vi "read_ini_file.vi"(8 "error in (no error)":errorcluster, 11 "configuration file path":path=path "D:/config.ini") -> (0 "error out":errorcluster, 1 "values":string[](array[string]), 2 "keys":string[](array[string]), 3 "sections":string[](array[string]))   [LabVIEW 2009]
uses:
  <vilib>/Utility/config.llb/Read Key (String).vi
  <vilib>/Utility/config.llb/NI_LVConfig.lvlib
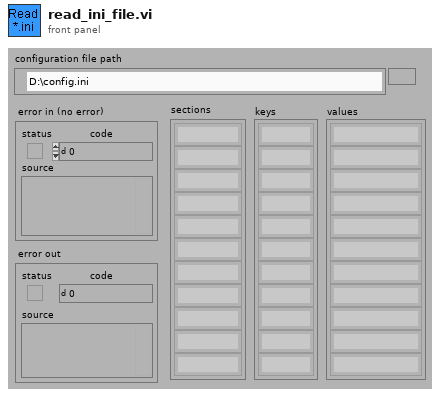
[diagram p1: front panel]
types:
  T1 = typedef "NI_LVConfig.lvlib/Config Data RefNum.ctl" = refnum<k1>
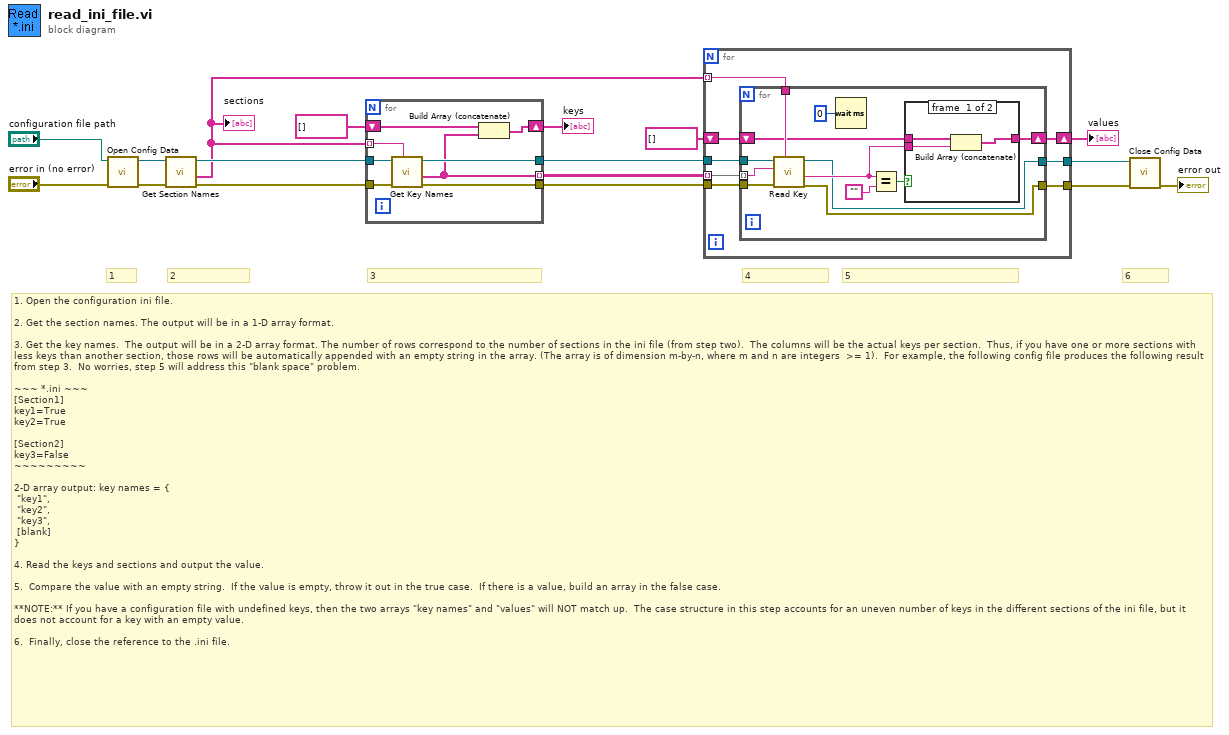
[diagram p0: block diagram]
diagram:
  # "1. Open the configuration ini file.\n\n2. Get the section names. The output will be in a 1-D array format.\n\n3. Get the key names.  The output will be in a 2-D array format. The number of rows correspond to the number of sections in the ini file (from step two).  The columns will be the actual keys per section.  Thus, if you have one or more sections with less keys than another section, those rows will be automatically appended with an empty string in the array. (The array is of dimension m-by-n, where m and n are integers  >= 1).  For example, the following config file produces the following result from step 3.  No worries, step 5 will address this \"blank space\" problem.\n\n~~~ *.ini ~~~\n[Section1]\nkey1=True\nkey2=True\n\n[Section2]\nkey3=False\n~~~~~~~~~\n\n2-D array output: key names = {\n \"key1\",\n \"key2\",\n \"key3\",\n [blank]\n}\n\n4. Read the keys and sections and output the value.\n\n5.  Compare the value with an empty string.  If the value is empty, throw it out in the true case.  If there is a value, build an array in the false case.\n\n**NOTE:** If you have a configuration file with undefined keys, then the two arrays \"key names\" and \"values\" will NOT match up.  The case structure in this step accounts for an uneven number of keys in the different sections of the ini file, but it does not account for a key with an empty value.\n\n6.  Finally, close the reference to the .ini file."
  # "6"
  # "5"
  # "4"
  # "3"
  # "2"
  # "1"
  n1 = call <vilib>:"Open Config Data.vi"("error in (no error)"="error in (no error)", "configuration file path"="configuration file path") -> ("error out"=w17:errorcluster, "refnum"=w16:T1)  [unwired: 7 in, 1 out]
  n2 = call <vilib>:"Get Section Names.vi"("error in (no error)"=w17, "refnum"=w16) -> ("error out"=w14:errorcluster, "section names"=w8:string[], "refnum out"=w15:T1)  [unwired: 7 in]
  "sections" <- w8
  n3 = for {
    tunnel: w15 -> [w25]
    tunnel: w14 -> [w24]
    tunnel: [w23] -> w9
    tunnel: [w22] -> w10
    tunnel: w8 -> [w21] mode=indexing
    shift-right: [w20] -> w6
    shift-left: string[] [] -> [w19]
    tunnel: [w18] -> w5 mode=indexing
    n4 = call <vilib>:"Get Key Names.vi"("section"=w21, "error in (no error)"=w24, "refnum"=w25) -> ("error out"=w23:errorcluster, "key names"=w18:string[], "refnum out"=w22:T1)  [unwired: 5 in, 1 out]
    n5 = Build Array (concatenate)(w19, w18) -> (w20:string[])
  }
  "keys" <- w6
  n6 = for {
    tunnel: w10 -> [w32]
    tunnel: w9 -> [w33]
    tunnel: w8 -> [w31] mode=indexing
    tunnel: w5 -> [w30] mode=indexing
    shift-right: [w29] -> w3
    shift-left: string[] [] -> [w28]
    tunnel: [w27] -> w2
    tunnel: [w26] -> w1
    n7 = for {
      tunnel: w32 -> [w43]
      tunnel: w31 -> [w45]
      tunnel: w30 -> [w42] mode=indexing
      tunnel: w33 -> [w41]
      shift-right: [w37] -> w29
      shift-left: w28 -> [w36]
      tunnel: [w35] -> w27
      tunnel: [w34] -> w26
      n8 = call-poly <vilib>:"Read Key.vi"("section"=w45, "error in (no error)"=w41, "key"=w42, "refnum"=w43) -> ("error out"=w34:errorcluster, "value"=w38:string, "refnum out"=w35:T1)  [unwired: 4 in, 1 out]
      n9 = Wait (ms)(milliseconds to wait=u32 0) -> ()  [unwired: 1 out]
      n10 = Equal?(x=w38, y="") -> (x = y?=w39:bool)
      n11 = case shown="False" w39 {
        tunnel: w38 -> [w48 _]
        tunnel: [w47 w49] -> w37
        tunnel: w36 -> [w46 w49]
        frame #0 {
          n12 = Build Array (concatenate)(w46, w48) -> (w47:string[])
        }
        frame #1 {
        }
      }
    }
  }
  "values" <- w3
  n13 = call <vilib>:"Close Config Data.vi"("error in (no error)"=w1, "refnum"=w2) -> ("error out"=→"error out":errorcluster)  [unwired: 8 in, 1 out]
